vi "ini_sesion.vi"(8 "error in (no error)":errorcluster, 11 "pulse_gen_and_detect_p2p in":refnum<class "pulse_gen_and_detect_p2p.lvclass">) -> (0 "error out":errorcluster, 3 "pulse_gen_and_detect_p2p out":refnum<class "pulse_gen_and_detect_p2p.lvclass">)   [LabVIEW 2021, in "pulse_gen_and_detect_p2p.lvclass"]
uses:
  pulse_gen_and_detect_p2p.lvclass
  pulse_gen_and_detect_p2p.lvclass/pulse_gen_and_detect_p2p.ctl
  <instrlib>/niRFSG/niRFSG.llb/niRFSG Ref Clock Sources.ctl
  <instrlib>/niRFSA/niRFSA.llb/niRFSA Acquisition Types.ctl
  <vilib>/FPGAPlugInAG/PXIe-5785 (KU060)/niLvFpga_Open_PXIe-5785 (KU060).vi
  <vilib>/rvi/interface/common/dynamic/niFpgaDynamicAddResources.vi
  <vilib>/FPGAPlugInAG/Dynamic/niLvFpga_P2PGetEndpoint_Dynamic.vi
  <vilib>/Utility/error.llb/Error Cluster From Error Code.vi
  <vilib>/rvi/interface/common/niFpgaWaitOnOcc.vi
  <vilib>/rvi/errors/niLvFpgaAdjustHostInterfaceError.vi
  <vilib>/rvi/interface/nirviOpenFPGA/nirviOpenFPGA.xnode
  FPGA Bitfiles/5785_p2p_IQ_gen_1_6GHz_max_and_pulse_detector.lvbitx
  <vilib>/rvi/interface/nirviMethod/nirviMethod.xnode
  <vilib>/rvi/interface/nirviReadWriteControl/nirviReadWriteControl.xnode
  <vilib>/rvi/errors/niLvFpgaMergeErrorWithErrorCode.vi
  <vilib>/FPGAPlugInAG/Dynamic/niLvFpga_StopFifo_Dynamic.vi
  <vilib>/FPGAPlugInAG/Dynamic/niLvFpga_ConfigureFifo_Dynamic.vi
  NiFpgaLv.dll
  <vilib>/rvi/interface/Simulation/niFpgaSimulationCallBeginRW.vi
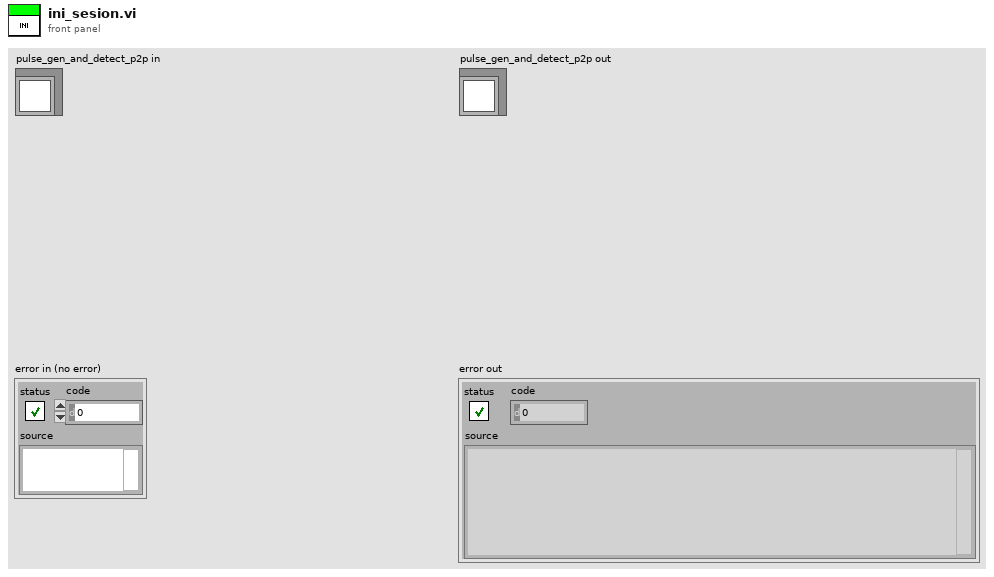
[diagram p1: front panel]
types:
  T1 = typedef "nirio_resource_hc.ctl" = tag
  T2 = cluster{"min PW (fft cycels)":u16, "max PW (fft cycels)":u16, "max gap (fft cycels)":u8, "detection bar (liniar amp)":fxp<+,64,63>, "peak detect":bool}
  T3 = enum16{"open", "open or create", "create or replace", "create", "open (read-only)"}
  T4 = typedef "niRFSG Ref Clock Sources.ctl" = string
  T5 = typedef "niRFSA Acquisition Types.ctl" = i32
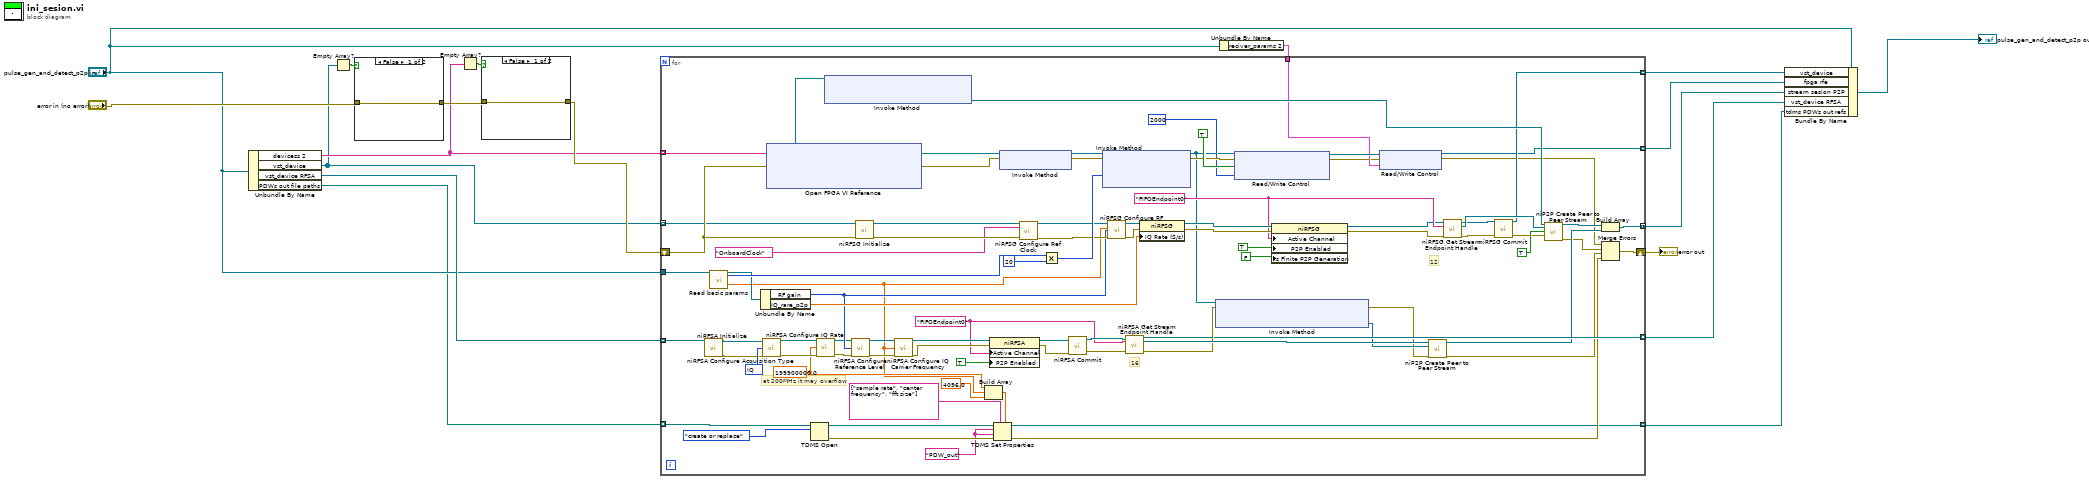
[diagram p0: block diagram]
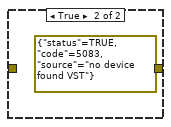
[diagram p2: hidden frame]
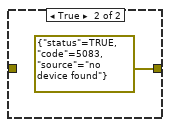
[diagram p3: hidden frame]
diagram:
  n1 = Unbundle By Name("pulse_gen_and_detect_p2p in") -> ("devicess 2"=w12:T1[], "vst_device"=w11:refnum<k15>[], "vst_device RFSA"=w7:refnum<k15>[], "PDWs out file paths"=w3:path[])
  n2 = Empty Array?(array=w11) -> (empty?=w17:bool)
  n3 = case shown="False" w17 {
    tunnel: [w19 errorcluster {"status"=TRUE, "code"=5083, "source"="no device found VST"} ("error in (no error)")] -> w16
    tunnel: "error in (no error)" -> [w19 _]
    frame False {
    }
    frame True {
    }
  }
  n4 = Empty Array?(array=w12) -> (empty?=w18:bool)
  n5 = case shown="False" w18 {
    tunnel: [w21 errorcluster {"status"=TRUE, "code"=5083, "source"="no device found"} ("error in (no error)")] -> w13
    tunnel: w16 -> [w21 _]
    frame False {
    }
    frame True {
    }
  }
  n6 = Unbundle By Name("pulse_gen_and_detect_p2p in") -> ("reciver_params 2"=w4:T2)
  n7 = for {
    tunnel: w12 -> [w74] mode=indexing
    tunnel: w11 -> [w23] mode=indexing
    tunnel: "pulse_gen_and_detect_p2p in" -> [w73]
    shift-right: [w26] -> w15
    shift-left: w13 -> [w75]
    tunnel: [w72] -> w10 mode=indexing
    tunnel: [w48] -> w9 mode=indexing
    tunnel: [w50] -> w8 mode=concatenating
    tunnel: w7 -> [w71] mode=indexing
    tunnel: [w55] -> w6 mode=indexing
    tunnel: w4 -> [w47]
    tunnel: w3 -> [w46] mode=indexing
    tunnel: [w25] -> w2 mode=indexing
    w32 = "PDW_out" ("group name")
    w36 = 199900000.0 ("IQ rate (S/s)")
    w24 = "FIFOEndpoint0" ("Active Channel")
    w70 = T5 100 items=["IQ"=100, "Spectrum"=101] ("acquisition type")
    w82 = "FIFOEndpoint0" ("format string")
    # "at 200MHz it may overflow"
    # "16"
    # "12"
    n8 = call <instrlib>:"niRFSA Initialize.vi"("resource name"=w71) -> ("instrument handle out"=w69:refnum<k15>, "error out"=w68:errorcluster)  [unwired: 13 in]
    n9 = call-dynamic "Read basic params.vi"("device_type in"=w73) -> ("device_type out"=w77:refnum<class "pulse_gen_and_detect_p2p.lvclass">, "buffer size"=w78:u32, "center frequency (Hz)"=w35:dbl)  [unwired: 13 in, 3 out]
    n10 = Unbundle By Name(w77) -> ("RF gain"=w67:i32, "IQ_rare_p2p"=w86:dbl)
    n11 = call <instrlib>:"niRFSA Configure Acquisition Type.vi"("instrument handle"=w69, "acquisition type"=w70, "error in"=w68) -> ("instrument handle out"=w42:refnum<k15>, "error out"=w39:errorcluster)  [unwired: 11 in]
    n12 = xnode "Open FPGA VI Reference"("error in"=w75, "resource name"=w74) -> ("FPGA VI Reference Out"=w96:refnum<k20>, "error out"=w105:errorcluster)
    n13 = TDMS Open(10:T3."create or replace" ("operation (0:open)"), 11:w46) -> (0:w43:errorcluster, 3:w44:refnum<k34>)  [unwired: 5 in]
    n14 = call <instrlib>:"niRFSA Configure IQ Rate.vi"("instrument handle"=w42, "IQ rate (S/s)"=w36, "error in"=w39) -> ("instrument handle out"=w41:refnum<k15>, "error out"=w40:errorcluster)  [unwired: 11 in]
    n15 = xnode "Invoke Method"("FPGA VI Reference In"=w96) -> ("Writer"=w76:refnum<k20>)  [unwired: 1 in, 2 out]
    n16 = call <instrlib>:"niRFSA Configure Reference Level.vi"("instrument handle"=w41, "reference level (dBm)"=w67, "error in"=w40) -> ("instrument handle out"=w66:refnum<k15>, "error out"=w65:errorcluster)  [unwired: 11 in]
    n17 = call <instrlib>:"niRFSG Initialize.vi"("resource name"=w23, "error in"=w75) -> ("instrument handle"=w100:refnum<k15>, "error out"=w99:errorcluster)  [unwired: 12 in]
    n18 = call <instrlib>:"niRFSA Configure IQ Carrier Frequency.vi"("instrument handle"=w66, "carrier frequency"=w35, "error in"=w65) -> ("instrument handle out"=w63:refnum<k15>, "error out"=w64:errorcluster)  [unwired: 11 in]
    n19 = Build Array(w36, w35, 4096.0 ("element")) -> (w33:dbl[])
    n20 = property class="niRFSA"(reference=w63, error in=w64, "Active Channel"=w24, "P2P Enabled"=TRUE ("Peer-to-Peer:Enabled")) -> (reference out=w62:refnum<k15>, error out=w61:errorcluster)
    n21 = TDMS Set Properties(5:w33, 7:string[] ["sample rate", "center frequency", "fft size"] ("property names"), 8:w43, 9:w32, 10:w32, 11:w44) -> (0:w30:errorcluster, 3:w25:refnum<k34>)  [unwired: 2 out]
    n22 = xnode "Invoke Method"("FPGA VI Reference In"=w96, "error in"=w105) -> ("FPGA VI Reference Out"=w103:refnum<k20>, "error out"=w104:errorcluster)
    n23 = call <instrlib>:"niRFSG Configure Ref Clock.vi"("instrument handle"=w100, "ref clock source"=T4 "OnboardClock", "error in"=w99) -> ("instrument handle out"=w92:refnum<k15>, "error out"=w91:errorcluster)  [unwired: 11 in]
    n24 = Multiply(x=w78, y=u32 20) -> (x*y=w107:u32)
    n25 = call <instrlib>:"niRFSA Commit.vi"("instrument handle"=w62, "error in"=w61) -> ("instrument handle out"=w60:refnum<k15>, "error out"=w59:errorcluster)  [unwired: 12 in]
    n26 = xnode "Invoke Method"("FPGA VI Reference In"=w103, "error in"=w104, "Requested Depth"=w107) -> ("FPGA VI Reference Out"=w57:refnum<k20>, "error out"=w101:errorcluster)  [unwired: 1 out]
    n27 = call <instrlib>:"niRFSG Configure RF.vi"("instrument handle"=w92, "frequency (Hz)"=w35, "power level (dBm)"=w67, "error in"=w91) -> ("instrument handle out"=w90:refnum<k15>, "error out"=w89:errorcluster)  [unwired: 10 in]
    n28 = call <instrlib>:"niRFSA Get Stream Endpoint Handle.vi"("instrument handle"=w60, "stream endpoint"=w24, "error in"=w59) -> ("instrument handle out"=w55:refnum<k15>, "writer handle"=w58:refnum<k20>, "error out"=w56:errorcluster)  [unwired: 10 in]
    n29 = property class="niRFSG"(reference=w90, error in=w89, "IQ Rate (S/s)"=w86) -> (reference out=w88:refnum<k15>, error out=w87:errorcluster)
    n30 = xnode "Invoke Method"("FPGA VI Reference In"=w57, "error in"=w56) -> ("error out"=w53:errorcluster, "Reader"=w54:refnum<k20>)  [unwired: 1 out]
    n31 = xnode "Read/Write Control"("FPGA VI Reference In"=w57, "error in"=w101, "reset system clock"=TRUE, "P2P empty room for runing"=u32 2000) -> ("FPGA VI Reference Out"=w49:refnum<k20>, "error out"=w31:errorcluster)
    n32 = property class="niRFSG"(reference=w88, error in=w87, "Active Channel"=w82, "P2P Enabled"=TRUE ("Peer-to-Peer:Enabled"), "Is Finite P2P Generation"=FALSE ("Peer-to-Peer:Is Finite Generation")) -> (reference out=w81:refnum<k15>, error out=w80:errorcluster)
    n33 = xnode "Read/Write Control"("FPGA VI Reference In"=w49, "error in"=w31, "reciver_params 2"=w47) -> ("FPGA VI Reference Out"=w48:refnum<k20>, "error out"=w27:errorcluster)
    n34 = call <vilib>:"niP2P Create Peer to Peer Stream.vi"("writer"=w58, "reader"=w54, "error in (no error)"=w53) -> ("stream session"=w51:refnum<k20>, "error out"=w29:errorcluster)  [unwired: 11 in]
    n35 = call <instrlib>:"niRFSG Get Stream Endpoint Handle.vi"("instrument handle"=w81, "stream endpoint"=w82, "error in"=w80) -> ("instrument handle out"=w85:refnum<k15>, "reader handle"=w97:refnum<k20>, "error out"=w84:errorcluster)  [unwired: 10 in]
    n36 = call <instrlib>:"niRFSG Commit.vi"("instrument handle"=w85, "error in"=w84) -> ("instrument handle out"=w72:refnum<k15>, "error out"=w83:errorcluster)  [unwired: 12 in]
    n37 = call <vilib>:"niP2P Create Peer to Peer Stream.vi"("writer"=w76, "reader"=w97, "enable stream (T)"=TRUE, "error in (no error)"=w83) -> ("stream session"=w52:refnum<k20>, "error out"=w28:errorcluster)  [unwired: 10 in]
    n38 = Build Array(w52, w51) -> (w50:refnum<k20>[])
    n39 = Merge Errors(w27, w28, w29, w30) -> (w26:errorcluster)
  }
  "error out" <- w15
  n40 = Bundle By Name(cluster="pulse_gen_and_detect_p2p in", "vst_device"=w10, "fpga rfe"=w9, "stream sesion P2P"=w8, "vst_device RFSA"=w6, "tdms PDWs out refs"=w2) -> (→"pulse_gen_and_detect_p2p out":refnum<class "pulse_gen_and_detect_p2p.lvclass">)
